vi "SCMP - print screen RT2.vi"(7 "mode (save)":enum16{"Init", "Save"}(ring)=enum."Save", 8 "error in (no error)":errorcluster, 10 "Source":string, 11 "FITS Header in":T1={"Wavelength (nm)"=530.15, "Exposure (s)"=0.05, "Tuning Delay (ms)"=200.0, "Beam Type (-1/1)"=1.0, "Tuning Voltages"=[1.111, 2.222, 3.333, 4.444], "Observer"="observer", "Light Shapping Diffuser"=enum."In Beam", "Comment"="", "Data Type"=enum."LIVE", "Mod Cycles"=1, "SCD Calibration Optics"=enum."1 - Polarizer @0, I+Q", "SCD Emission Line Filter"=enum."1-557.6nm", "Cookbook"="", "COMP-S Calibration Wheel"=enum."Dark", "COMP-S Andover Filter Wheel"=enum."530.3nm/HWB 0.34nm (Fe XIV)", "FOV Rotation (deg)"=66.0, "Objective Lens Position (mm)"=0.0, "Occulter size"=0.0, "Time End"=timestamp(3382374145.421875 s since 1904-01-01), "Acc Exposure (s)"=0.0, "Time Stamp Array"=[], "Camera Serial Number"=[], "Camera Temp"=[], "Camera PI (mm)"=[0.0, 0.0, 0.0], "Time Start"=timestamp(3382374145.421875 s since 1904-01-01), "Peripherals"={"ILX controler"=FALSE, "Zone temperatures"=FALSE, "Andor"=FALSE, "Andor 2"=FALSE, "PI Stages"=FALSE, "AISAS mechanisms"=FALSE, "AISAS Mech.lvclass"=refnum, "Zone temp ref"=variant, "FWs"=FALSE}, "FITS paths"=[], "Cameras"=enum."Andor", "load preset cbk"=FALSE, "periodic check count"=0, "COMP-S Calibration Wheel 2"=enum."Dark", "Calib"=enum."Dark", "Abso Aperture"=66.0, "Nominal Aperture"=66.0, "Pointer IP"="127.0.0.1"} {"Nominal Aperture" format="%.1f"; "Abso Aperture" format="%.1f"; "Camera PI (mm)" format="%_3g"; "Acc Exposure (s)" format="%^.3g"; "Occulter size" format="%.2f"; "Objective Lens Position (mm)" min=70.0 max=152.0 format="%.2f"; "FOV Rotation (deg)" format="%.1f"; "Exposure (s)" format="%^.3g"; "Wavelength (nm)" format="%_6g"}) -> (0 "error out":errorcluster, 3 "FITS Header out":T1={"Wavelength (nm)"=0.0, "Exposure (s)"=0.0, "Tuning Delay (ms)"=0.0, "Beam Type (-1/1)"=0.0, "Tuning Voltages"=[], "Observer"="", "Light Shapping Diffuser"=enum."Out of Beam", "Comment"="", "Data Type"=enum."LIVE", "Mod Cycles"=0, "SCD Calibration Optics"=enum."1 - Polarizer @0, I+Q", "SCD Emission Line Filter"=enum."1-557.6nm", "Cookbook"="", "COMP-S Calibration Wheel"=enum."Dark", "COMP-S Andover Filter Wheel"=enum."530.3nm/HWB 0.34nm (Fe XIV)", "FOV Rotation (deg)"=0.0, "Objective Lens Position (mm)"=0.0, "Occulter size"=0.0, "Time End"=timestamp(0 s since 1904-01-01), "Acc Exposure (s)"=0.0, "Time Stamp Array"=[], "Camera Serial Number"=[], "Camera Temp"=[], "Camera PI (mm)"=[], "Time Start"=timestamp(0 s since 1904-01-01), "Peripherals"={"ILX controler"=FALSE, "Zone temperatures"=FALSE, "Andor"=FALSE, "Andor 2"=FALSE, "PI Stages"=FALSE, "AISAS mechanisms"=FALSE, "AISAS Mech.lvclass"=refnum, "Zone temp ref"=variant, "FWs"=FALSE}, "FITS paths"=[], "Cameras"=enum."Andor", "load preset cbk"=FALSE, "periodic check count"=0, "COMP-S Calibration Wheel 2"=enum."Dark", "Calib"=enum."Dark", "Abso Aperture"=66.0, "Nominal Aperture"=66.0, "Pointer IP"="127.0.0.1"} {"Nominal Aperture" format="%.1f"; "Abso Aperture" format="%.1f"; "Camera PI (mm)" format="%_3g"; "Acc Exposure (s)" format="%^.3g"; "Occulter size" format="%.2f"; "Objective Lens Position (mm)" min=70.0 max=152.0 format="%.2f"; "FOV Rotation (deg)" format="%.1f"; "Exposure (s)" format="%^.3g"; "Wavelength (nm)" format="%_6g"})   [LabVIEW 2014]
uses:
  Controls/SCD - FITS Cluster.ctl
  AISAS/Mech/AISAS Mech.lvclass
  AISAS/Controls/Diffuser.ctl
  Controls/FITS Data type.ctl
  Controls/SCD - Calibration Optics Filter Wheel.ctl
  Controls/SCD - EDT - Emission Line Filter Wheel.ctl
  Controls/CoMP-S Controls/Polarization Optics Filter Wheel.ctl
  Controls/CoMP-S Controls/Emission Line Filter Wheel.ctl
  AISAS/Controls/focus.ctl
  Controls/peripherals.ctl
  Controls/Cameras select.ctl
  <vilib>/Utility/sysdir.llb/System Directory Type.ctl
  System.Windows.Forms
  System.Drawing
  Controls/Globals.vi
panel:
  out "printsreen path":path
  out "file name":string
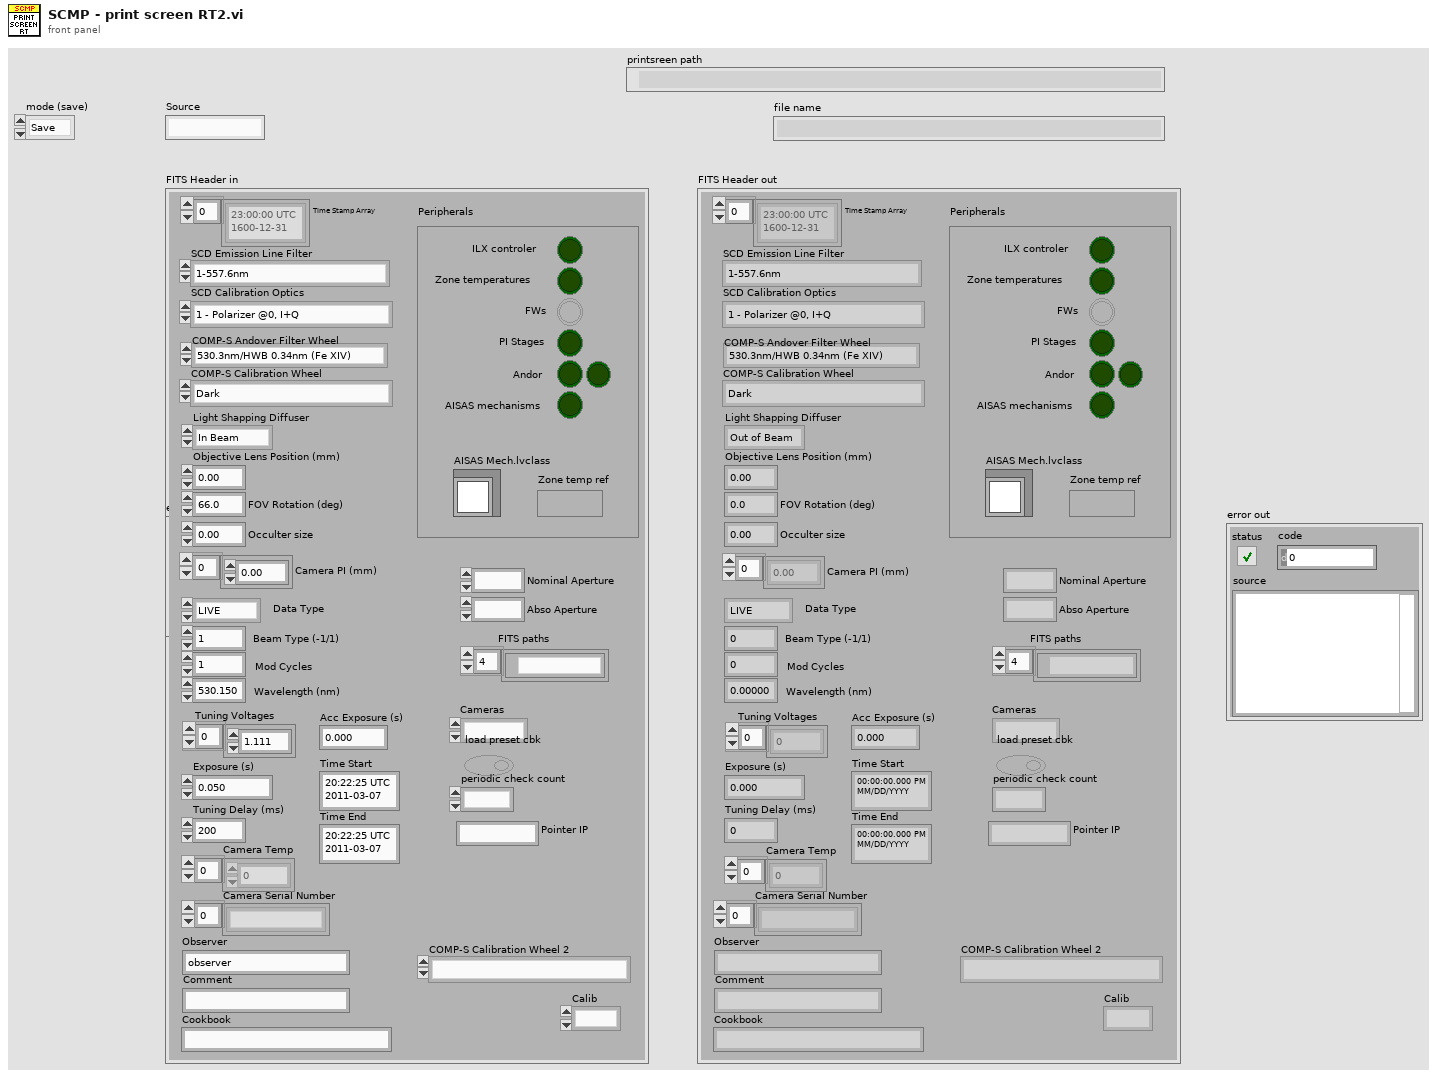
[diagram p1: front panel]
types:
  T1 = typedef "SCD - FITS Cluster.ctl" = cluster{"Wavelength (nm)":dbl, "Exposure (s)":dbl, "Tuning Delay (ms)":dbl, "Beam Type (-1/1)":dbl, "Tuning Voltages":dbl[], "Observer":string, "Light Shapping Diffuser":T2, "Comment":string, "Data Type":T3, "Mod Cycles":u16, "SCD Calibration Optics":T4, "SCD Emission Line Filter":T5, "Cookbook":string, "COMP-S Calibration Wheel":T6, "COMP-S Andover Filter Wheel":T7, "FOV Rotation (deg)":dbl, "Objective Lens Position (mm)":T8, "Occulter size":dbl, "Time End":timestamp, "Acc Exposure (s)":dbl, "Time Stamp Array":timestamp[], "Camera Serial Number":string[], "Camera Temp":dbl[], "Camera PI (mm)":dbl[], "Time Start":timestamp, "Peripherals":T9, "FITS paths":path[], "Cameras":T10, "load preset cbk":bool, "periodic check count":i32, "COMP-S Calibration Wheel 2":T6, "Calib":enum16{"Dark", "Flat"}, "Abso Aperture":dbl, "Nominal Aperture":dbl, "Pointer IP":string}
  T2 = typedef "Diffuser.ctl" = enum16{"Out of Beam", "In Beam"}
  T3 = typedef "FITS Data type.ctl" = enum16{"LIVE", "DARK", "FLAT", "CALI", "OBSE", "ABSO", "AURE", "TARG", "OBJE", "HOLE", "OREX", "THRO", "CHIP"}
  T4 = typedef "SCD - Calibration Optics Filter Wheel.ctl" = enum16{"1 - Polarizer @0, I+Q", "2 - Polarizer @90, I-Q", "3 - Polarizer @45, I+U", "4 - Polarizer @135, I-U", "5 - Polarizer @0, Retarder @45, I+V", "6 - Polarizer @0, Retarder @135, I-V", "7 - Dark", "8 - Clear", "9 - N/A"}
  T5 = typedef "SCD - EDT - Emission Line Filter Wheel.ctl" = enum16{"1-557.6nm", "2-587.6nm", "3-589.6nm", "4-630.2nm", "5-656.4nm", "6-849.8nm", "7-854.2nm", "8-866.2nm", "9-1083.0nm"}
  T6 = typedef "Polarization Optics Filter Wheel.ctl" = enum16{"Dark", "Clear", "Exchange Lens", "Polarizer @0, I+Q", "Polarizer @90, I-Q", "Polarizer @45, I+U", "Polarizer @135, I-U", "Polarizer @0, Retarder @45, I+V", "Polarizer @0, Retarder @135, I-V"}
  T7 = typedef "Emission Line Filter Wheel.ctl" = enum16{"530.3nm/HWB 0.34nm (Fe XIV)", "587.6nm/HBW 0.44nm (He I D3)", "637.5nm/HBW 0.53nm (Fe X)", "656.3nm/HBW 0.57nm (H-Alpha)", "789.2nm/HBW 0.85nm (Fe XI)", "854.2nm/HBW 1.01nm (Ca I)", "1074.7nm/HBW 2.34nm (Fe XIII)", "1079.8nm/HBW 1.64nm (Fe XIII)", "1083.0nm/HBW 1.66nm (He I)"}
  T8 = typedef "focus.ctl" = dbl
  T9 = typedef "peripherals.ctl" = cluster{"ILX controler":bool, "Zone temperatures":bool, "Andor":bool, "Andor 2":bool, "PI Stages":bool, "AISAS mechanisms":bool, "AISAS Mech.lvclass":refnum<class "AISAS Mech.lvclass">, "Zone temp ref":variant, "FWs":bool}
  T10 = typedef "Cameras select.ctl" = enum16{"Andor", "GDR"}
  T11 = enum16{"Left Mouse Button", "Right Mouse Button", "Ctrl-Break", "Middle Mouse Button (3-button mice only)", "X1 mouse button (Win2k Only)", "X2 Mouse Button (Win2k Only)", "Undefined (1)", "BACKSPACE", "TAB", "Reserved (1)", "Reserved (2)", "CLEAR", "ENTER", "Undefined (2)", "Undefined (3)", "SHIFT", "CTRL", "ALT", "PAUSE", "CAPS LOCK", "IME Kana mode", "Undefined (4)", "IME Junja mode", "IME final mode", "IME Hanja mode", "IME Kanji mode", "Undefined    ", "ESC", "IME convert", "IME nonconvert", "IME accept", "IME mode change request", "SPACEBAR", "PAGE UP", "PAGE DOWN", "END", "HOME", "LEFT ARROW", "UP ARROW", "RIGHT ARROW", "DOWN ARROW", "SELECT", "PRINT", "EXECUTE", "PRINT SCREEN", "INS", "DEL", "HELP"}
  T12 = typedef "System Directory Type.ctl" = i32
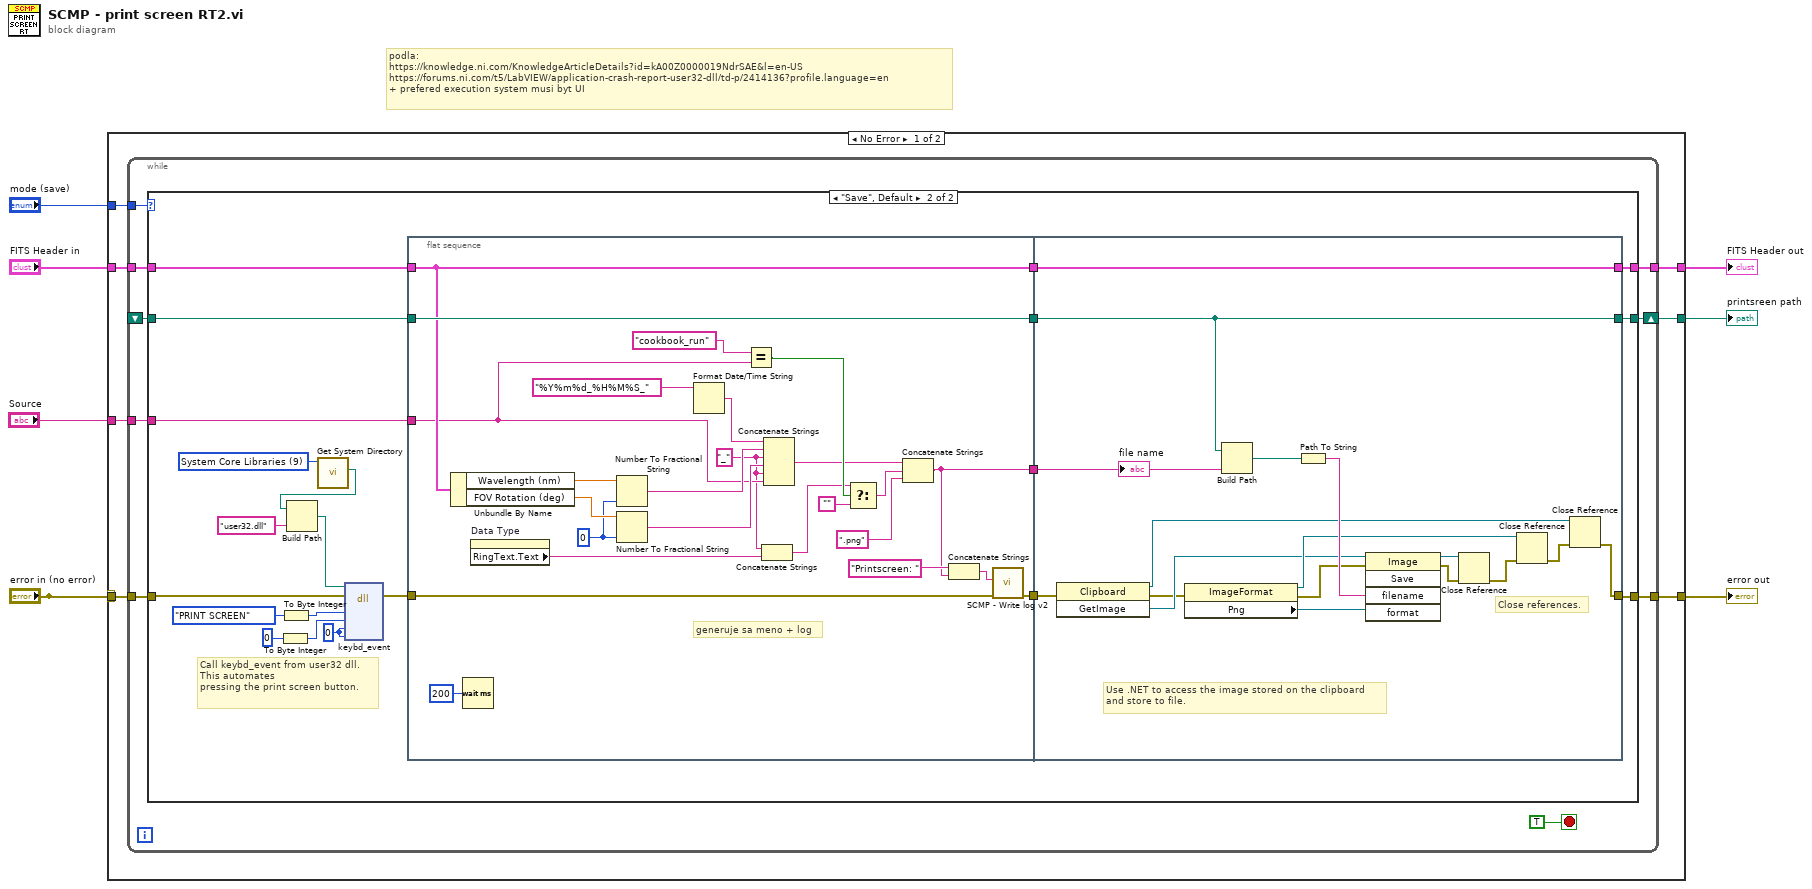
[diagram p0: block diagram]
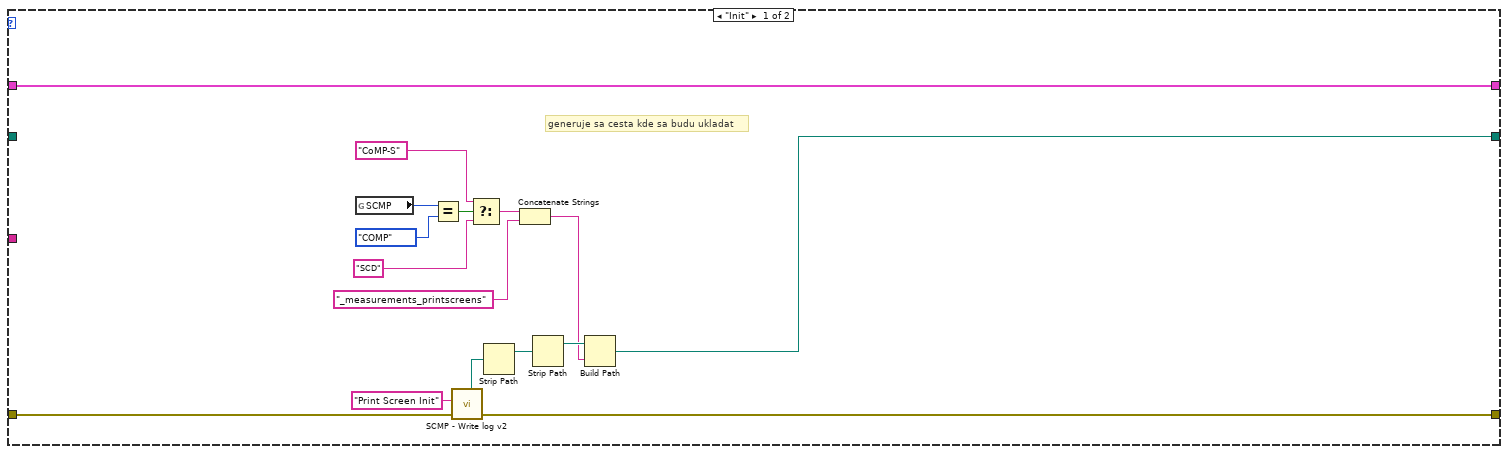
[diagram p2: hidden frame]
diagram:
  # "podla: \nhttps://knowledge.ni.com/KnowledgeArticleDetails?id=kA00Z0000019NdrSAE&l=en-US\nhttps://forums.ni.com/t5/LabVIEW/application-crash-report-user32-dll/td-p/2414136?profile.language=en\n+ prefered execution system musi byt UI"
  n1 = case shown="No Error" "error in (no error)" {
    selector: "error in (no error)" -> [w13 w104]
    tunnel: "error in (no error)" -> [_ _]
    tunnel: [w10 w103] -> w7
    tunnel: "FITS Header in" -> [w12 w103]
    tunnel: [w11 w104] -> w5
    tunnel: "mode (save)" -> [w14 _]
    tunnel: [w9 _] -> w2
    tunnel: "Source" -> [w8 _]
    frame No Error {
      n2 = while {
        tunnel: w14 -> [w22]
        tunnel: w13 -> [w21]
        shift-right: [w20] -> w9
        shift-left: _ -> [w19]
        tunnel: w12 -> [w18]
        tunnel: [w17] -> w11
        tunnel: [w16] -> w10
        tunnel: w8 -> [w15]
        stop <- TRUE stop-if-true
        n3 = case shown="\"Save\", Default" w22 {
          tunnel: w21 -> [w39 w49]
          tunnel: [w34 w57] -> w20
          tunnel: w19 -> [_ w58]
          tunnel: w18 -> [w24 w60]
          tunnel: [w25 w59] -> w17
          tunnel: [w24 w56] -> w16
          tunnel: w15 -> [_ w44]
          frame "Init" {
            # "generuje sa cesta kde sa budu ukladat"
            n4 = global read "Globals.vi" "SCMP"() -> (w33:enum16{"COMP", "SCD"})
            n5 = Equal?(x=w33, y=enum16{"COMP", "SCD"}."COMP") -> (x = y?=w31:bool)
            n6 = call "SCMP - Write log v2.vi"("Error to log"=w39, "data"="Print Screen Init") -> ("error out"=w25:errorcluster, "Today's SCMP Log File"=w37:path)  [unwired: 7 in, 1 out]
            n7 = Select(t="CoMP-S" ("name or relative path"), s=w31, f="SCD" ("name or relative path")) -> (s? t:f=w28:string)
            n8 = Strip Path(path=w37) -> (stripped path=w36:path)  [unwired: 1 out]
            n9 = Concatenate Strings(w28, "_measurements_printscreens" ("name or relative path")) -> (w26:string)
            n10 = Strip Path(path=w36) -> (stripped path=w35:path)  [unwired: 1 out]
            n11 = Build Path(base path=w35, name or relative path=w26) -> (appended path=w34:path)
          }
          frame "Save", Default {
            w48 = T12 9 items=["User Home"=0, "User Desktop"=1, "User Documents"=2, "User Application Data"=3, "User Preferences"=4, "User Temporary"=5, "Public Documents"=6, "Public Application Data"=7, "Public Preferences"=8, "Public Cache"=13, "System Core Libraries"=9, "System Installed Libraries"=10, "Application Files"=11, "Boot Volume Root"=12] ("system directory type")
            w51 = 0 ("Input Value")
            # "Call keybd_event from user32 dll.  This automates\npressing the print screen button."
            n12 = To Byte Integer(number=i16 0) -> (8bit integer=w53:i8)
            n13 = To Byte Integer(number=T11."PRINT SCREEN" ("Keyboard Stroke")) -> (8bit integer=w55:i8)
            n14 = call <vilib>:"Get System Directory.vi"("system directory type"=w48) -> ("system directory"=w47:path)  [unwired: 10 in]
            n15 = Build Path(base path=w47, name or relative path="user32.dll") -> (appended path=w46:path)
            n16 = dll-call lib="C:/Windows/System32/user32.dll" fn="keybd_event"(path in=w46, error in=w49, w55, w53, w51, w51) -> (error out=w50:errorcluster)  [unwired: 6 in, 1 out]
            n17 = flat-sequence {
              tunnel: w60 -> [w75]
              tunnel: w58 -> [w76]
              tunnel: w50 -> [w74]
              tunnel: [w77] -> w43
              tunnel: [w76] -> w42
              tunnel: [w75] -> w41
              tunnel: w44 -> [w72]
              tunnel: [w61] -> w40
              tunnel: [w95] -> w59
              tunnel: w43 -> [w92]
              tunnel: w42 -> [w88]
              tunnel: w41 -> [w94]
              tunnel: [w88] -> w57
              tunnel: [w94] -> w56
              tunnel: w40 -> [w86]
              frame #0 {
                w70 = "_" ("string")
                w80 = i16 0 ("precision (6)")
                # "generuje sa meno + log"
                n18 = Unbundle By Name(w75) -> ("Wavelength (nm)"=w78:dbl, "FOV Rotation (deg)"=w81:dbl)
                n19 = Wait (ms)(milliseconds to wait=u32 200) -> ()  [unwired: 1 out]
                n20 = property on="Data Type" class="Enum (strict)"() -> ("RingText.Text"=w71:string)  [unwired: 2 in, 2 out]
                n21 = Number To Fractional String(number=w78, precision (6)=w80) -> (F-format string=w79:string)  [unwired: 2 in]
                n22 = Number To Fractional String(number=w81, precision (6)=w80) -> (F-format string=w82:string)  [unwired: 2 in]
                n23 = Format Date/Time String(time format string (%c)="%Y%m%d_%H%M%S_") -> (date/time string=w84:string)  [unwired: 2 in]
                n24 = Equal?(x="cookbook_run" ("Source"), y=w72) -> (x = y?=w66:bool)
                n25 = Concatenate Strings(w70, w71) -> (w64:string)
                n26 = Concatenate Strings(w84, w79, w70, w82, w70, w72) -> (w65:string)
                n27 = Select(t=w64, s=w66, f="") -> (s? t:f=w68:string)
                n28 = Concatenate Strings(w65, w68, ".png" ("time format string (%c)")) -> (w61:string)
                n29 = Concatenate Strings("Printscreen: " ("data"), w61) -> (w63:string)
                n30 = call "SCMP - Write log v2.vi"("Error to log"=w74, "data"=w63) -> ("error out"=w77:errorcluster)  [unwired: 7 in, 2 out]
              }
              frame #1 {
                # "Close references."
                # "Use .NET to access the image stored on the clipboard\nand store to file."
                n31 = invoke class="Clipboard" method="GetImage"(error in=w92) -> (reference out=w89:refnum<k24>, error out=w90:errorcluster, "GetImage"=w91:refnum<k24>)  [unwired: 2 in]
                n32 = property class="ImageFormat"(error in=w90) -> (reference out=w98:refnum<k24>, error out=w96:errorcluster, "Png"=w93:refnum<k24>)  [unwired: 1 in]
                n33 = Build Path(base path=w88, name or relative path=w86) -> (appended path=w87:path)
                n34 = Path To String(path=w87) -> (string=w102:string)
                n35 = invoke class="Image" method="Save"(reference=w91, error in=w96, "filename"=w102, "format"=w93) -> (reference out=w100:refnum<k24>, error out=w101:errorcluster)  [unwired: 1 in, 3 out]
                n36 = Close Reference(reference=w100, error in (no error)=w101) -> (error out=w99:errorcluster)
                n37 = Close Reference(reference=w98, error in (no error)=w99) -> (error out=w97:errorcluster)
                n38 = Close Reference(reference=w89, error in (no error)=w97) -> (error out=w95:errorcluster)
                "file name" <- w86
              }
            }
          }
        }
      }
    }
    frame Error {
    }
  }
  "FITS Header out" <- w7
  "error out" <- w5
  "printsreen path" <- w2
